vi "_extractWaveform.vi"(0 "Waveforms":waveform(dbl)[](array[waveform]), 1 "Event Object In":string[](array[string]), 2 "Starting Index":u32[](array[numeric]), 3 "error in (no error)":errorcluster) -> (7 "Event Object Out":string[](array[string]), 10 "error out":errorcluster)   [LabVIEW 2019]
uses:
  <vilib>/JDP Science/JSONtext/support/Format JSON Object.vi
  <vilib>/JDP Science/JSONtext/Get all Object Items.vi
  <vilib>/JDP Science/JSONtext/Set Multiple Object Items.vi
  <vilib>/JDP Science/JSONtext/JSONtext.lvlib
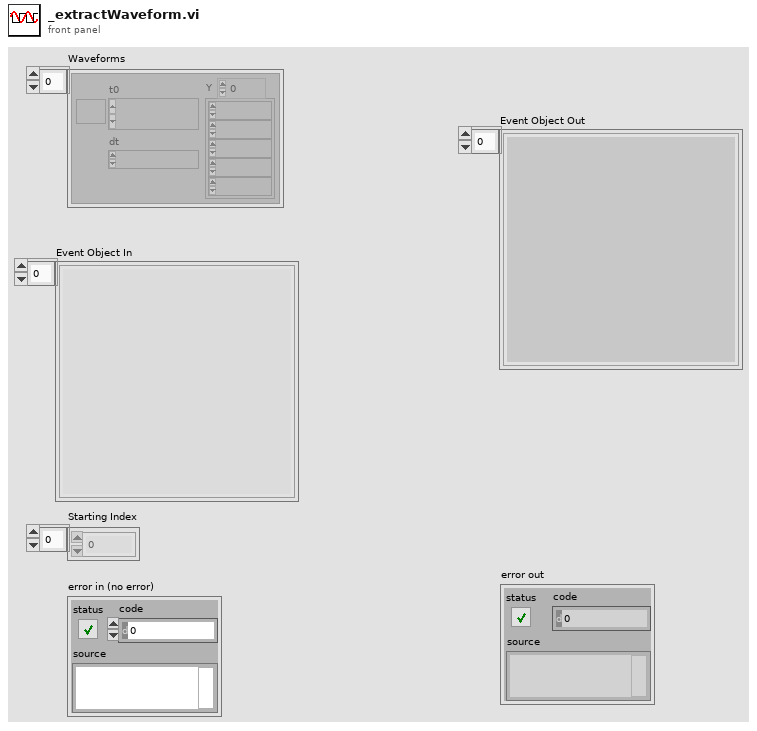
[diagram p1: front panel]
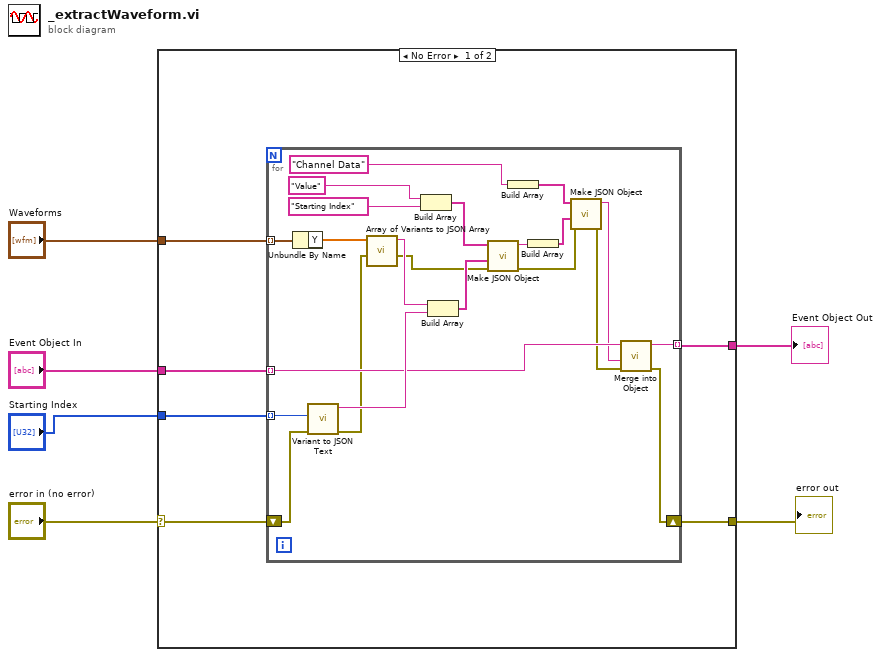
[diagram p0: block diagram]
diagram:
  n1 = case shown="No Error" "error in (no error)" {
    selector: "error in (no error)" -> [w12 w35]
    tunnel: "Waveforms" -> [w11 _]
    tunnel: "Event Object In" -> [w10 w36]
    tunnel: "Starting Index" -> [w9 _]
    tunnel: [w8 w36] -> w3
    tunnel: [w7 w35] -> w2
    frame No Error {
      n2 = for {
        shift-right: [w20] -> w7
        shift-left: w12 -> [w23]
        tunnel: w11 -> [w34] mode=indexing
        tunnel: w10 -> [w25] mode=indexing
        tunnel: w9 -> [w28] mode=indexing
        tunnel: [w24] -> w8 mode=indexing
        n3 = Unbundle By Name(w34) -> ("Y"=w32:dbl[])
        n4 = call <vilib>:"Variant to JSON Text.vi"("error in (no error)"=w23, "Variant"=w28) -> ("error out"=w22:errorcluster, "<JSON>"=w27:string)  [unwired: 7 in, 1 out]
        n5 = call <vilib>:"Array of Variants to JSON Array.vi"("error in (no error)"=w22, "Array of Variants"=w32) -> ("error out"=w21:errorcluster, "<JSON>"=w29:string)  [unwired: 8 in]
        n6 = Build Array("Value", "Starting Index") -> (w30:string[])
        n7 = Build Array(w29, w27) -> (w26:string[])
        n8 = call <vilib>:"Make JSON Object.vi"("error in (no error)"=w21, "JSON Items"=w26, "Item Names"=w30) -> ("error out"=w15:errorcluster, "<JSON>"=w17:string)  [unwired: 7 in]
        n9 = Build Array("Channel Data") -> (w18:string[])
        n10 = Build Array(w17) -> (w16:string[])
        n11 = call <vilib>:"Make JSON Object.vi"("error in (no error)"=w15, "JSON Items"=w16, "Item Names"=w18) -> ("error out"=w14:errorcluster, "<JSON>"=w13:string)  [unwired: 7 in]
        n12 = call <vilib>:"Merge into Object.vi"("error in (no error)"=w14, "JSON Object to Merge"=w13, "JSON"=w25) -> ("error out"=w20:errorcluster, "<JSON>"=w24:string)  [unwired: 6 in]
      }
    }
    frame Error {
    }
  }
  "Event Object Out" <- w3
  "error out" <- w2
